vi "test_Open UDP connection using Initialize node.vi"(8 "error in (no error)":errorcluster, 11 "TestCase in":refnum<class "Instrument Addon Ethernet Protocol Unit Tests.lvclass">) -> (0 "error out":errorcluster, 3 "TestCase out":refnum<class "Instrument Addon Ethernet Protocol Unit Tests.lvclass">)   [LabVIEW 2023, in "Instrument Addon Ethernet Protocol Unit Tests.lvclass"]
uses:
  Instrument Addon Ethernet Protocol Unit Tests.lvclass
  <vilib>/addons/_JKI Toolkits/VI Tester/TestCase.llb/TestCase.lvclass
  UDP/UDP.lvclass
  Constants.vi
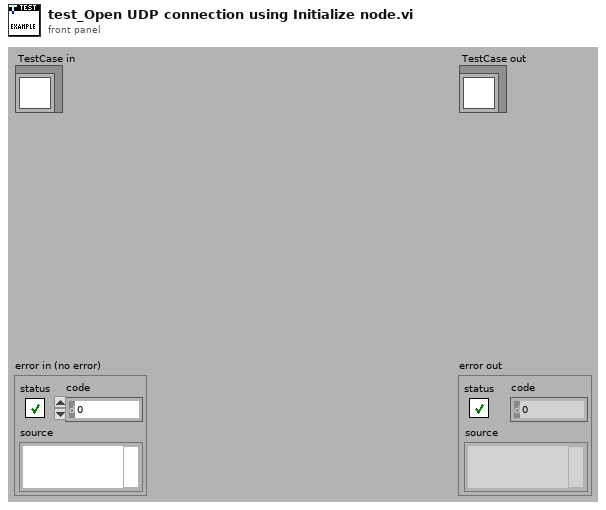
[diagram p1: front panel]
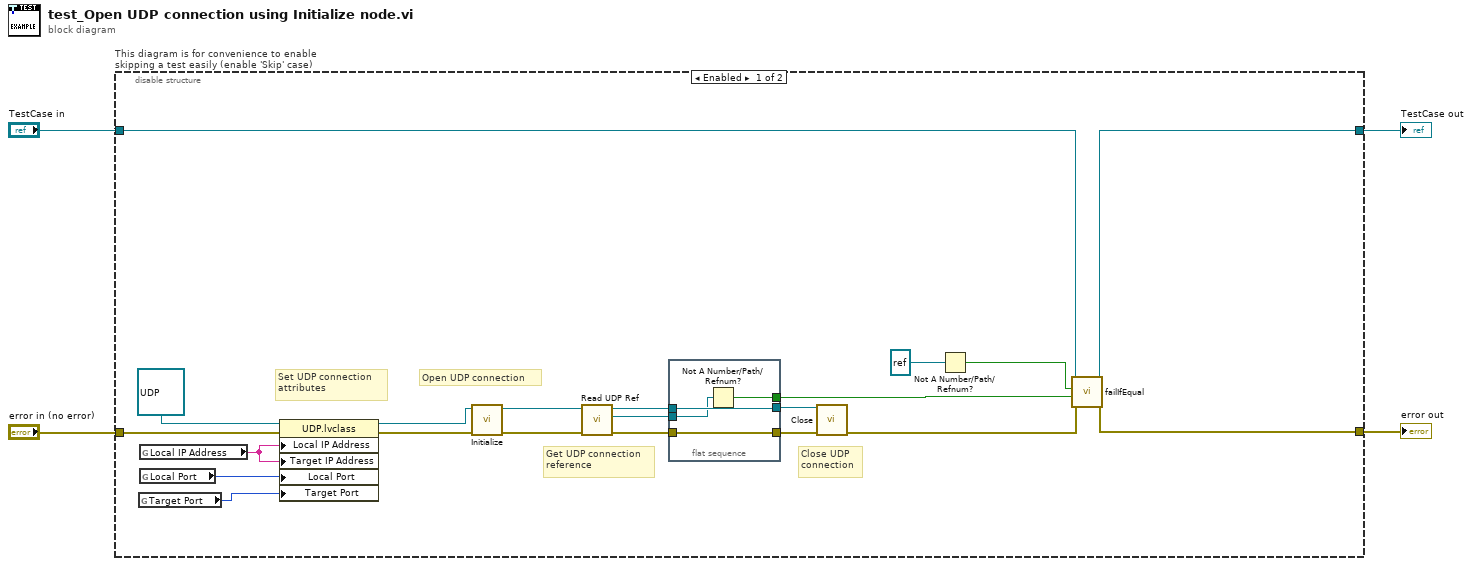
[diagram p0: block diagram]
diagram:
  n1 = disable-structure "This diagram is for convenience to enable skipping a test easily (enable 'Skip' case)" shown="Enabled" {
    disable-tunnel: "TestCase in" -> [w25 w33]
    disable-tunnel: [w24 w31] -> w1
    disable-tunnel: [w23 w32] -> w3
    disable-tunnel: "error in (no error)" -> [w21 w30]
    frame Enabled {
      # "Close UDP \nconnection"
      # "Get UDP connection\nreference"
      # "Open UDP connection"
      # "Set UDP connection \nattributes"
      n2 = global read "Constants.vi" "Target Port"() -> (w11:u16)
      n3 = global read "Constants.vi" "Local IP Address"() -> (w13:string)
      n4 = global read "Constants.vi" "Local Port"() -> (w12:u16)
      n5 = property class="UDP.lvclass"(reference=refnum<class "UDP.lvclass"> refnum ("Protocols.lvlib:UDP.lvclass"), error in=w21, "Local IP Address"=w13, "Target IP Address"=w13, "Local Port"=w12, "Target Port"=w11) -> (reference out=w16:refnum<class "UDP.lvclass">, error out=w17:errorcluster)
      n6 = call-dynamic "Initialize.vi"("error in (no error)"=w17, "UDP in"=w16) -> ("error out"=w15:errorcluster, "UDP out"=w14:refnum<class "UDP.lvclass">)  [unwired: 8 in]
      n7 = call "Read UDP Ref.vi"("error in (no error)"=w15, "UDP in"=w14) -> ("error out"=w8:errorcluster, "UDP Ref"=w10:refnum<k16>, "UDP out"=w9:refnum<class "UDP.lvclass">)  [unwired: 7 in]
      n8 = flat-sequence {
        tunnel: w10 -> [w26]
        tunnel: w9 -> [w28]
        tunnel: w8 -> [w29]
        tunnel: [w29] -> w7
        tunnel: [w28] -> w6
        tunnel: [w27] -> w5
        frame #0 {
          n9 = Not A Number/Path/Refnum?(number/path/refnum=w26) -> (NaN/Path/Refnum?=w27:bool)
        }
      }
      n10 = call-dynamic "Close.vi"("error in (no error)"=w7, "UDP in"=w6) -> ("error out"=w20:errorcluster)  [unwired: 8 in, 1 out]
      n11 = Not A Number/Path/Refnum?(number/path/refnum=refnum<k16> refnum ("UDP Ref")) -> (NaN/Path/Refnum?=w18:bool)
      n12 = call-dynamic "failIfEqual.vi"("error in (no error)"=w20, "y"=w5, "x"=w18, "TestCase in"=w25) -> ("error out"=w23:errorcluster, "TestCase out"=w24:refnum<class "Instrument Addon Ethernet Protocol Unit Tests.lvclass">)  [unwired: 6 in]
    }
    frame Disabled {
      # "skip test result while test is under development"
      n13 = call <vilib>:"skip.vi"("error in (no error)"=w30, "TestCase in"=w33) -> ("error out"=w32:errorcluster, "TestCase out"=w31:refnum<class "Instrument Addon Ethernet Protocol Unit Tests.lvclass">)  [unwired: 8 in]
    }
  }
  "error out" <- w3
  "TestCase out" <- w1
